vi "Update Coefficients.vi"(8 "error in (no error)":errorcluster, 10 "coeffs":dbl[](array[numeric]), 11 "references":T1) -> (0 "error out":errorcluster)   [LabVIEW 2013, in "Polynomial Scale editor node.lvclass"]
uses:
  Polynomial Scale editor node.lvclass
  <vilib>/NI/DCAF Table API/Table Manager/object ref.ctl
  <vilib>/NI/DCAF/Tag Editor Core/Configuration Editor/Classes/Engine Parent/Engine Parent Editor Node.lvclass
  <vilib>/NI/DCAF/Tag Editor Core/Configuration Editor/Classes/Module editor node/module editor node.lvclass
  module/configuration/Polynomial Scale configuration.lvclass
  <vilib>/NI/DCAF Templates/DCAF Scaling/editor node/Scaling editor node.lvclass
  <vilib>/NI/DCAF Templates/DCAF Scaling/editor node/Scaling editor node.lvclass/Scaling editor node.ctl
  <vilib>/NI/DCAF Templates/DCAF Scaling/editor node/accessors/Read active scale index .vi
  <vilib>/NI/DCAF Table API/Table Manager/Table Manager.lvclass
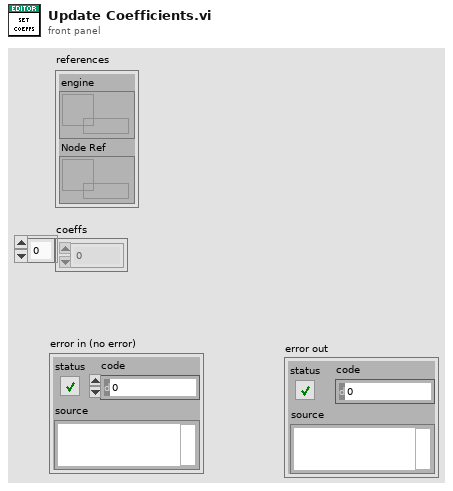
[diagram p1: front panel]
types:
  T1 = typedef "Table Manager.lvlib/Table Manager.lvclass/object ref.ctl" = cluster{"engine":refnum<data-value>, "Node Ref":refnum<data-value>}
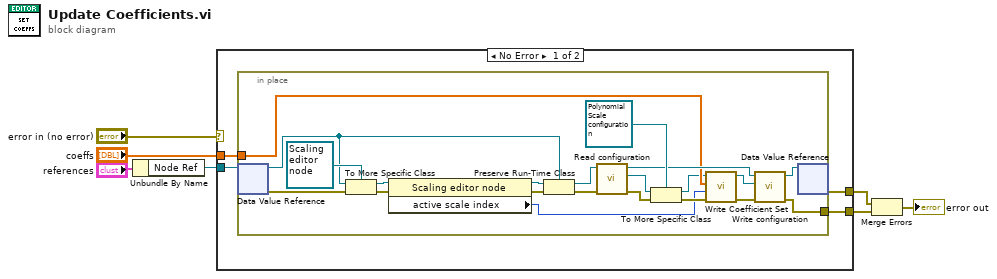
[diagram p0: block diagram]
diagram:
  n1 = Unbundle By Name("references") -> ("Node Ref"=w1:refnum<data-value>)
  n2 = case shown="No Error" "error in (no error)" {
    selector: "error in (no error)" -> [_ w33]
    tunnel: "coeffs" -> [w11 _]
    tunnel: [w10 w33] -> w5
    tunnel: [w9 _] -> w4
    tunnel: w1 -> [w8 _]
    frame No Error {
      n3 = in-place {
        in-place-border: w11 -> [w25]
        in-place-border: [w28] -> w9
        n4 = in-place-dvr #1(w8) -> (w18:refnum<class "module editor node.lvclass">, w20:errorcluster)
        n5 = To More Specific Class(target class=refnum<class "Scaling editor node.lvclass"> refnum ("Scaling editor node"), reference=w18, error in=w20) -> (specific class reference=w22:refnum<class "Scaling editor node.lvclass">, error out=w21:errorcluster)
        n6 = property class="Scaling editor node"(reference=w22, error in=w21) -> (reference out=w19:refnum<class "Scaling editor node.lvclass">, error out=w15:errorcluster, "active scale index "=w14:i32)
        n7 = Preserve Run-Time Class(object in=w19, error in=w15, 2:w18) -> (object out=w12:refnum<class "module editor node.lvclass">, error out=w24:errorcluster)
        n8 = call-dynamic "Read configuration.vi"("error in"=w24, "NISE_CEF_serializable node in"=w12) -> ("error out"=w31:errorcluster, "configuration"=w32:refnum<class "NISE_CEF_serializable configuration.lvclass">, "NISE_CEF_serializable node out"=w29:refnum<class "module editor node.lvclass">)  [unwired: 7 in]
        n9 = To More Specific Class(target class=refnum<class "Polynomial Scale configuration.lvclass"> refnum ("Polynomial Scale configuration"), reference=w32, error in=w31) -> (specific class reference=w17:refnum<class "Polynomial Scale configuration.lvclass">, error out=w16:errorcluster)
        n10 = call "Write Coefficient Set.vi"("error in (no error)"=w16, "scale index"=w14, "Coefficients"=w25, "Polynomial Scale configuration in"=w17) -> ("error out"=w26:errorcluster, "Polynomial Scale configuration out"=w27:refnum<class "Polynomial Scale configuration.lvclass">)  [unwired: 6 in]
        n11 = call-dynamic "Write configuration.vi"("error in"=w26, "configuration"=w27, "NISE_CEF_serializable node in"=w29) -> ("error out"=w28:errorcluster, "NISE_CEF_serializable node out"=w13:refnum<class "module editor node.lvclass">)  [unwired: 7 in]
        n12 = in-place-dvr #1(w13) -> (w10:errorcluster)  [unwired: 1 out]
      }
    }
    frame Error {
    }
  }
  n13 = Merge Errors(w5, w4) -> (→"error out":errorcluster)
